vi "VICI_10 mport_switch_pair.vi"(2 "Go to position":string="3", 4 "Valve COM":refnum<visa-resource-name>="COM8") -> (0 "Current position":string)   [LabVIEW 2023]
panel:
  out "error out":errorcluster
  out "read buffer":string
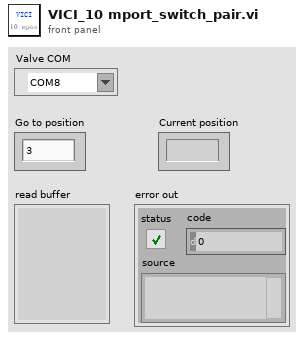
[diagram p1: front panel]
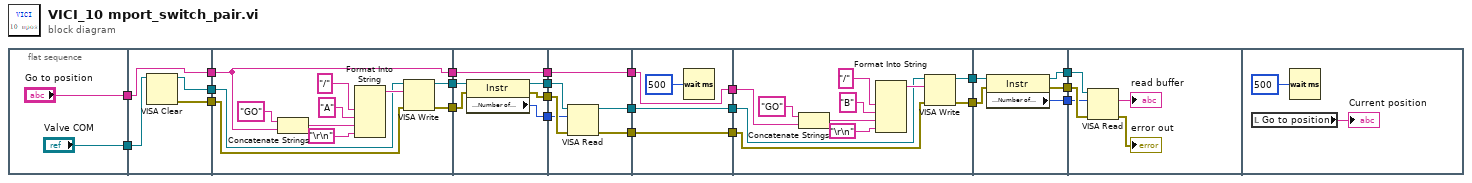
[diagram p0: block diagram]
diagram:
  n1 = flat-sequence {
    tunnel: ["Valve COM"] -> w20
    tunnel: ["Go to position"] -> w18
    tunnel: w20 -> [w29]
    tunnel: [w27] -> w19
    tunnel: w18 -> [w28]
    tunnel: [w28] -> w17
    tunnel: [w26] -> w16
    tunnel: w19 -> [w33]
    tunnel: w17 -> [w34]
    tunnel: [w34] -> w15
    tunnel: [w32] -> w14
    tunnel: [w31] -> w13
    tunnel: w16 -> [w30]
    tunnel: w15 -> [w46]
    tunnel: [w46] -> w12
    tunnel: w14 -> [w45]
    tunnel: [w43] -> w10
    tunnel: w13 -> [w44]
    tunnel: [w42] -> w8
    tunnel: [w41] -> w6
    tunnel: w12 -> [w52]
    tunnel: [w52] -> w11
    tunnel: w10 -> [w51]
    tunnel: [w48] -> w9
    tunnel: w8 -> [w50]
    tunnel: [w47] -> w7
    tunnel: w6 -> [w49]
    tunnel: w11 -> [w56]
    tunnel: [w56] -> w23
    tunnel: w9 -> [w55]
    tunnel: [w55] -> w22
    tunnel: w7 -> [w54]
    tunnel: [w54] -> w21
    tunnel: w23 -> [w64]
    tunnel: w22 -> [w60]
    tunnel: w21 -> [w59]
    tunnel: [w58] -> w5
    tunnel: [w57] -> w4
    tunnel: w5 -> [w72]
    tunnel: w4 -> [w71]
    tunnel: [w70] -> w3
    tunnel: [w69] -> w2
    tunnel: [w68] -> w1
    tunnel: w3 -> [w77]
    tunnel: w2 -> [w76]
    tunnel: w1 -> [w75]
    frame #0 {
    }
    frame #1 {
      n2 = VISA Clear(VISA resource name=w29) -> (VISA resource name out=w27:refnum<visa-resource-name>, error out=w26:errorcluster)  [unwired: 1 in]
    }
    frame #2 {
      n3 = Concatenate Strings("GO" ("input 3"), w34) -> (w36:string)
      n4 = Format Into String("/", "A" ("input 2"), w36, "\r\n") -> (resulting string=w38:string)  [unwired: 3 in, 1 out]
      n5 = VISA Write(VISA resource name=w33, write buffer=w38, error in (no error)=w30) -> (VISA resource name out=w32:refnum<visa-resource-name>, error out=w31:errorcluster)  [unwired: 1 out]
    }
    frame #3 {
      n6 = property class="Instr"(reference=w45, error in=w44) -> (reference out=w43:refnum<visa-resource-name>, error out=w42:errorcluster, "Serial Settings:Number of Bytes at Serial Port"=w41:u32)
    }
    frame #4 {
      n7 = VISA Read(VISA resource name=w51, byte count=w49, error in (no error)=w50) -> (VISA resource name out=w48:refnum<visa-resource-name>, error out=w47:errorcluster)  [unwired: 2 out]
    }
    frame #5 {
      n8 = Wait (ms)(milliseconds to wait=u32 500) -> ()  [unwired: 1 out]
    }
    frame #6 {
      n9 = Concatenate Strings("GO" ("input 3"), w64) -> (w66:string)
      n10 = Format Into String("/", "B" ("input 2"), w66, "\r\n") -> (resulting string=w67:string)  [unwired: 3 in, 1 out]
      n11 = VISA Write(VISA resource name=w60, write buffer=w67, error in (no error)=w59) -> (VISA resource name out=w58:refnum<visa-resource-name>, error out=w57:errorcluster)  [unwired: 1 out]
    }
    frame #7 {
      n12 = property class="Instr"(reference=w72, error in=w71) -> (reference out=w70:refnum<visa-resource-name>, error out=w69:errorcluster, "Serial Settings:Number of Bytes at Serial Port"=w68:u32)
    }
    frame #8 {
      n13 = VISA Read(VISA resource name=w77, byte count=w75, error in (no error)=w76) -> (read buffer=→"read buffer":string, error out=→"error out":errorcluster)  [unwired: 2 out]
    }
    frame #9 {
      n14 = local read "Go to position"() -> (→"Current position":string)
      n15 = Wait (ms)(milliseconds to wait=u32 500) -> ()  [unwired: 1 out]
    }
  }
